vi "state_select.vi"(9 "Mail":dbl, 10 "Curernt State":string) -> (2 "New State":string)   [LabVIEW 2016]
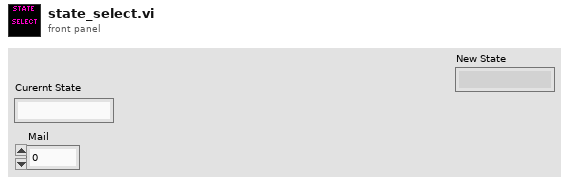
[diagram p1: front panel]
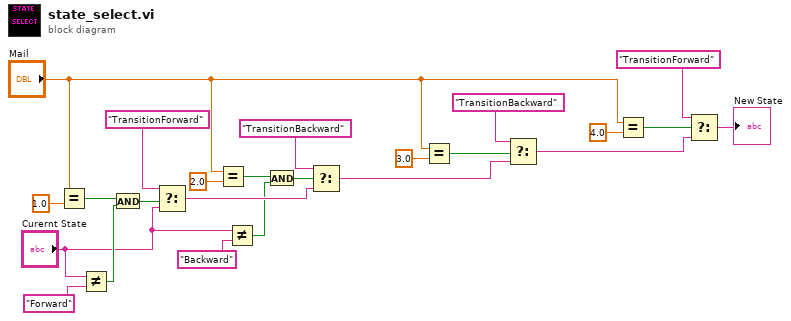
[diagram p0: block diagram]
diagram:
  n1 = Equal?(x="Mail", y=1.0) -> (x = y?=w8:bool)
  n2 = Not Equal?(x="Curernt State", y="Forward") -> (x != y?=w6:bool)
  n3 = And(x=w8, y=w6) -> (x .and. y?=w7:bool)
  n4 = Select(t="TransitionForward", s=w7, f="Curernt State") -> (s? t:f=w23:string)
  n5 = Equal?(x="Mail", y=2.0) -> (x = y?=w2:bool)
  n6 = Not Equal?(x="Curernt State", y="Backward") -> (x != y?=w1:bool)
  n7 = And(x=w2, y=w1) -> (x .and. y?=w3:bool)
  n8 = Select(t="TransitionBackward", s=w3, f=w23) -> (s? t:f=w21:string)
  n9 = Equal?(x="Mail", y=3.0) -> (x = y?=w14:bool)
  n10 = Select(t="TransitionBackward", s=w14, f=w21) -> (s? t:f=w19:string)
  n11 = Equal?(x="Mail", y=4.0) -> (x = y?=w12:bool)
  n12 = Select(t="TransitionForward", s=w12, f=w19) -> (s? t:f=→"New State":string)
